vi "CRYOLR.vi"(0 "Start Freq [Hz]":dbl=300.0 format="%.2f", 1 "Stop Freq [Hz]":dbl=3300.0 format="%.2f", 2 "Freq. Response [Hz,dB]":cluster{dbl, dbl}[](array[cluster])=[{200.0, -54.0}, {500.0, -51.0}, {1000.0, -48.0}, {2000.0, -49.0}, {4000.0, -60.0}] {"?" format="%.2f"; "?" format="%.2f"}, 3 "Exponent":dbl=2.2 format="%.3f", 4 "dB Correction [dB]":dbl format="%.2f") -> (5 "OLR [dB]":dbl=-9.801581591071972 format="%.2f")   [LabVIEW 2013]
panel:
  # "This VI calculates the average of the Freq. Response from Start Freq to Stop Freq. \nThe average is taken of the amplitude raised to the power of (1/Exponent).\nFreq. Response must be given ïn dB. The average is calculated using the trapezoid rule. Values for Freq. Response at exactly Start Freq and Stop Freq are found by interpolation.\n\nTo calculate OLR according to ANSI/IEEE 661, Start Freq must be 300 Hz and Stop Freq 3300 Hz, Exponent 2.2. Freq. Response shall (according to the std.) cover this freq. range and include at least 12 measurement points within the freq. range.\n\ndB Correction is added to Freq. Response, and may be used to correct for different dB references (e.g. if Freq. Response is dB rel 1 V/Pa and the OLR shall be dB rel 1 mV/Pa, the dB Correction shall be 60 dB).\n\nThe VI can use any Freq. Response with at least one point."
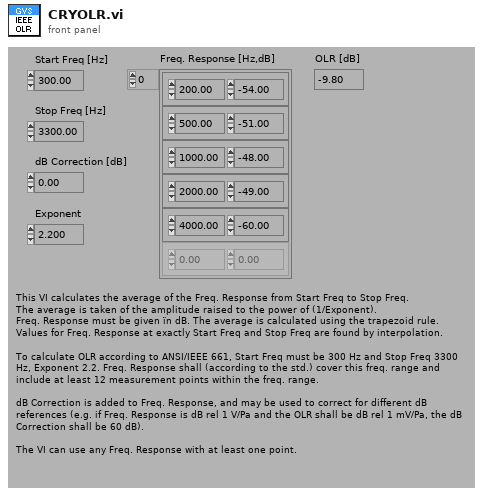
[diagram p1: front panel]
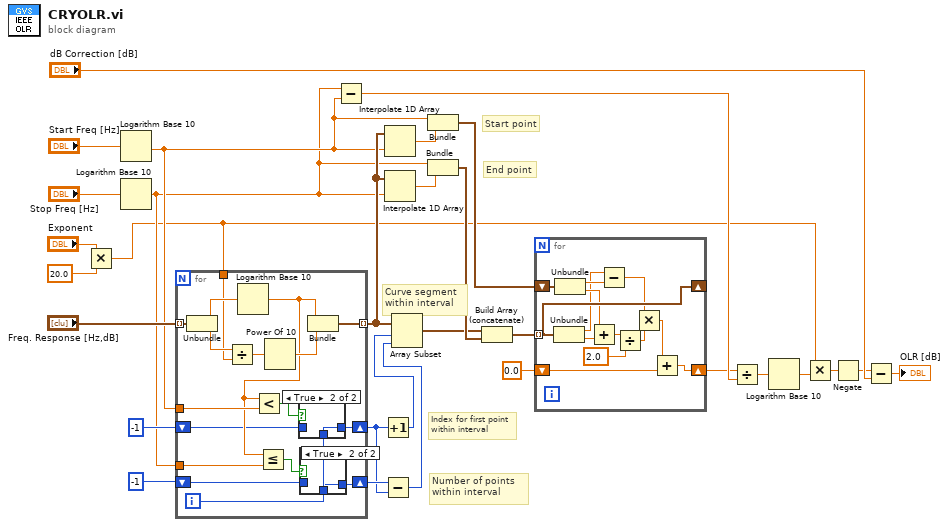
[diagram p0: block diagram]
diagram:
  # "End point"
  # "Curve segment \nwithin interval"
  # "Start point"
  # "Number of points \nwithin interval"
  # "Index for first point\nwithin interval"
  n1 = Multiply(x="Exponent", y=20.0) -> (x*y=w4:dbl)
  n2 = Logarithm Base 10(1:"Start Freq [Hz]") -> (0:w11:dbl)
  n3 = Logarithm Base 10(1:"Stop Freq [Hz]") -> (0:w10:dbl)
  n4 = for {
    tunnel: "Freq. Response [Hz,dB]" -> [w47] mode=indexing
    tunnel: [w43] -> w22 mode=indexing
    tunnel: w4 -> [w41]
    shift-right: [w32] -> w13
    shift-left: -1 -> [w35]
    shift-right: [w33] -> w19
    shift-left: -1 -> [w34]
    tunnel: w10 -> [w40]
    tunnel: w11 -> [w39]
    i -> [w31]
    n5 = Unbundle(w47) -> (w45:dbl, w46:dbl)
    n6 = Divide(x=w46, y=w41) -> (x/y=w44:dbl)
    n7 = Logarithm Base 10(1:w45) -> (0:w38:dbl)
    n8 = Less?(x=w38, y=w39) -> (x < y?=w37:bool)
    n9 = Less Or Equal?(x=w38, y=w40) -> (x <= y?=w36:bool)
    n10 = Power Of 10(x=w44) -> (10^x=w42:dbl)
    n11 = case shown="True" w37 {
      tunnel: w35 -> [w50 _]
      tunnel: [w50 w51] -> w32
      tunnel: w31 -> [_ w51]
      frame False {
      }
      frame True {
      }
    }
    n12 = case shown="True" w36 {
      tunnel: w34 -> [w48 _]
      tunnel: [w48 w49] -> w33
      tunnel: w31 -> [_ w49]
      frame False {
      }
      frame True {
      }
    }
    n13 = Bundle(w38, w42) -> (w43:cluster{dbl, dbl})  [unwired: 1 out]
  }
  n14 = Subtract(x=w10, y=w11) -> (x-y=w9:dbl)
  n15 = Increment(x=w13) -> (x+1=w18:i32)
  n16 = Subtract(x=w19, y=w13) -> (x-y=w12:i32)
  n17 = Interpolate 1D Array(1:w11, 2:w22) -> (0:w24:dbl)
  n18 = Interpolate 1D Array(1:w10, 2:w22) -> (0:w23:dbl)
  n19 = Array Subset(array=w22, index=w18, length=w12) -> (w25:cluster{dbl, dbl}[])
  n20 = Bundle(w11, w24) -> (w15:cluster{dbl, dbl})  [unwired: 1 out]
  n21 = Bundle(w10, w23) -> (w26:cluster{dbl, dbl})  [unwired: 1 out]
  n22 = Build Array (concatenate)(w25, w26) -> (w17:cluster{dbl, dbl}[])
  n23 = for {
    tunnel: w17 -> [w64] mode=indexing
    shift-right: [w64] -> _
    shift-left: w15 -> [w63]
    shift-right: [w56] -> w8
    shift-left: 0.0 -> [w57]
    n24 = Unbundle(w64) -> (w59:dbl, w61:dbl)
    n25 = Unbundle(w63) -> (w60:dbl, w62:dbl)
    n26 = Add(x=w62, y=w61) -> (x+y=w53:dbl)
    n27 = Subtract(x=w59, y=w60) -> (x-y=w58:dbl)
    n28 = Divide(x=w53, y=2.0) -> (x/y=w52:dbl)
    n29 = Multiply(x=w58, y=w52) -> (x*y=w55:dbl)
    n30 = Add(x=w55, y=w57) -> (x+y=w56:dbl)
  }
  n31 = Divide(x=w8, y=w9) -> (x/y=w7:dbl)
  n32 = Logarithm Base 10(1:w7) -> (0:w6:dbl)
  n33 = Multiply(x=w4, y=w6) -> (x*y=w5:dbl)
  n34 = Negate(x=w5) -> (-x=w1:dbl)
  n35 = Subtract(x=w1, y="dB Correction [dB]") -> (x-y=→"OLR [dB]":dbl)
